vi "Assert Wrapper.vi"(6 "error code (1)":i32=1, 7 "Label":string, 8 "error in (no error)":errorcluster, 11 "Assert?":bool) -> (0 "error out":errorcluster)   [LabVIEW 2009, in "Caraya.lvlib" / "Assert.lvclass"]
uses:
  Assert.lvclass
  Assert Factory/Assert Factory.lvclass
  Assert Factory Global/Assert Factory Global.lvclass
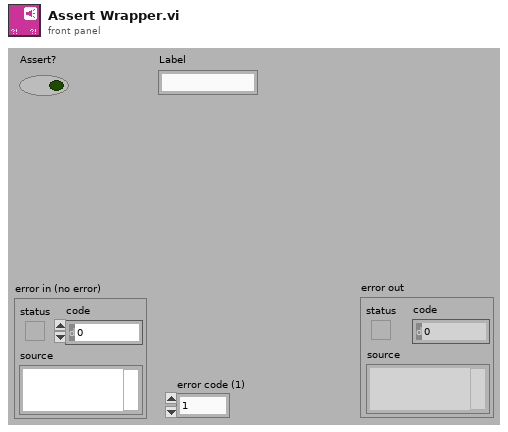
[diagram p1: front panel]
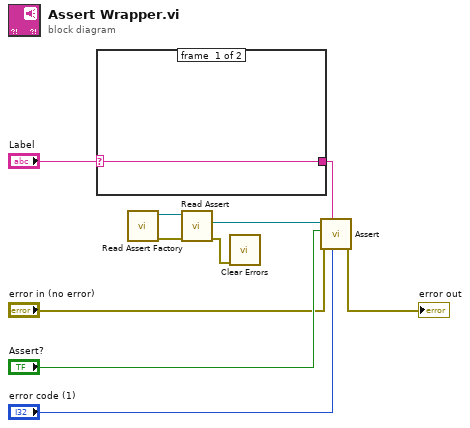
[diagram p0: block diagram]
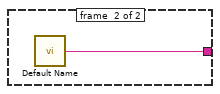
[diagram p2: hidden frame]
diagram:
  n1 = case shown="\"\"" "Label" {
    selector: "Label" -> [w11 _]
    tunnel: [w11 w12] -> w1
    frame #0 {
    }
    frame #1 {
      n2 = call "Default Name.vi"() -> ("String"=w12:string)
    }
  }
  n3 = call "Read Assert Factory.vi"() -> ("error out"=w6:errorcluster, "Assert Factory"=w8:refnum<class "Assert Factory.lvclass">)  [unwired: 10 in]
  n4 = call-dynamic "Read Assert.vi"("error in (no error)"=w6, "Assert Factory in"=w8) -> ("error out"=w3:errorcluster, "Assert"=w7:refnum<class "Assert.lvclass">)  [unwired: 7 in, 1 out]
  n5 = call <vilib>:"Clear Errors.vi"("error in (no error)"=w3) -> ()  [unwired: 6 in, 1 out]
  n6 = call-dynamic "Assert.vi"("error code (1)"="error code (1)", "Name"=w1, "error in (no error)"="error in (no error)", "Assert?"="Assert?", "Assert in"=w7) -> ("error out"=→"error out":errorcluster)  [unwired: 5 in, 1 out]
